vi "SUB VI desencriptador.vi"(8 "error in (no error)":errorcluster, 10 "PASSWORD":bool[](array[boolean]), 11 "Image 2":T1) -> (0 "error out":errorcluster, 3 "Image":T1(plugin-control))   [LabVIEW 2023]
uses:
  <vilib>/vision/Image Controls.llb/IMAQ Image.ctl
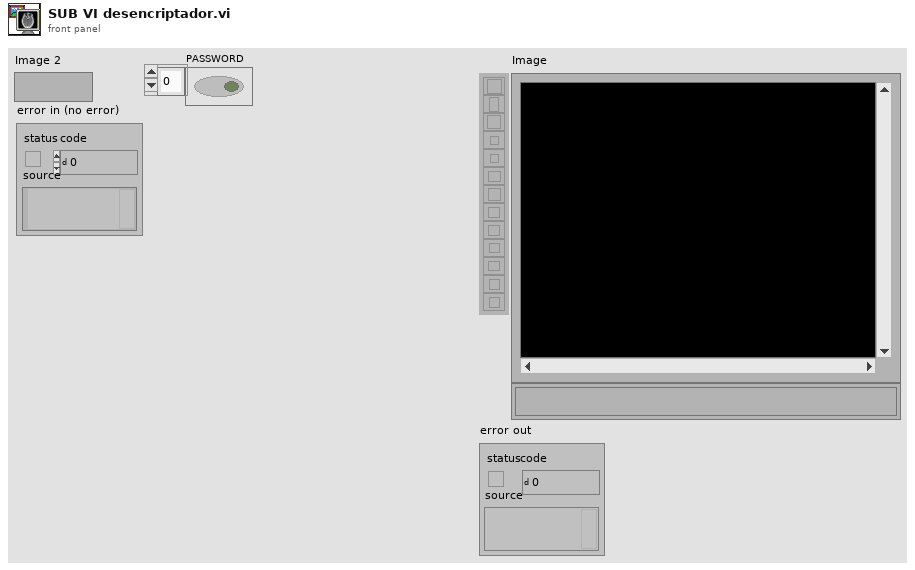
[diagram p1: front panel]
types:
  T1 = typedef "IMAQ Image.ctl" = refnum<image>
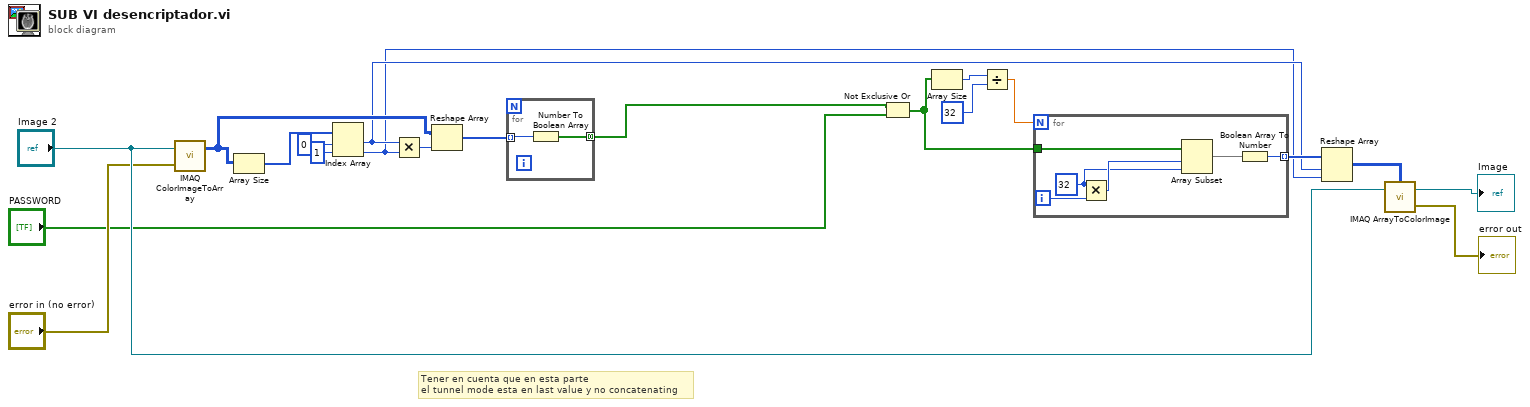
[diagram p0: block diagram]
diagram:
  # "Tener en cuenta que en esta parte \nel tunnel mode esta en last value y no concatenating"
  n1 = call "IMAQ ColorImageToArray"("Image"="Image 2", "error in (no error)"="error in (no error)") -> ("Image Pixels (U32)"=w17:u32[][])  [unwired: 2 in, 2 out]
  n2 = Array Size(array=w17) -> (size(s)=w20:i32[])
  n3 = Index Array(array=w20, index #1=0 ("index"), index #2=1 ("index")) -> (element #1=w8:i32, element #2=w7:i32)
  n4 = Multiply(x=w8, y=w7) -> (x*y=w16:i32)
  n5 = Reshape Array(w17, w16) -> (w15:u32[])
  n6 = for {
    tunnel: w15 -> [w22] mode=indexing
    tunnel: [w21] -> w14 mode=concatenating
    n7 = Number To Boolean Array(number=w22) -> (Boolean array=w21:bool[])
  }
  n8 = Not Exclusive Or(1:"PASSWORD", 2:w14) -> (0:w10:bool[])
  n9 = Array Size(array=w10) -> (size(s)=w13:i32)
  n10 = Divide(x=w13, y=32) -> (x/y=w11:dbl)
  n11 = for {
    N: w11 -> [_]
    tunnel: w10 -> [w28]
    tunnel: [w23] -> w9 mode=indexing
    i -> [w27]
    w25 = 32
    n12 = Multiply(x=w25, y=w27) -> (x*y=w26:i32)
    n13 = Array Subset(array=w28, index=w26, length=w25) -> (w24:bool[])
    n14 = Boolean Array To Number(Boolean array=w24) -> (number=w23:u32)
  }
  n15 = Reshape Array(w9, w8, w7) -> (w6:u32[][])
  n16 = call "IMAQ ArrayToColorImage"("Image Pixels (U32)"=w6, "Image"="Image 2") -> ("Image Out"=→"Image":T1, "error out"=→"error out":errorcluster)  [unwired: 3 in]
